vi "TimeLoop.vi"(4 "N":i32=100, 7 "Loop durations in":dbl[][](array[numeric])) -> (0 "Average fps":dbl, 3 "Loop durations out":dbl[][](array[numeric]))   [LabVIEW 2013]
doc: "Calculate average loop frequency over the last N (default: 100) iterations.\n\nMostly used for debugging"
uses:
  <vilib>/Analysis/baseanly.llb/Mean (DBL).vi
  <vilib>/Analysis/NI_AALBase.lvlib
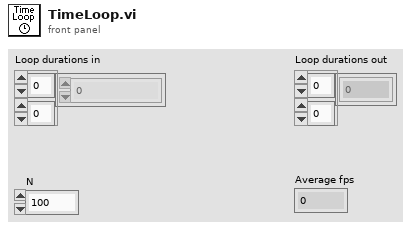
[diagram p1: front panel]
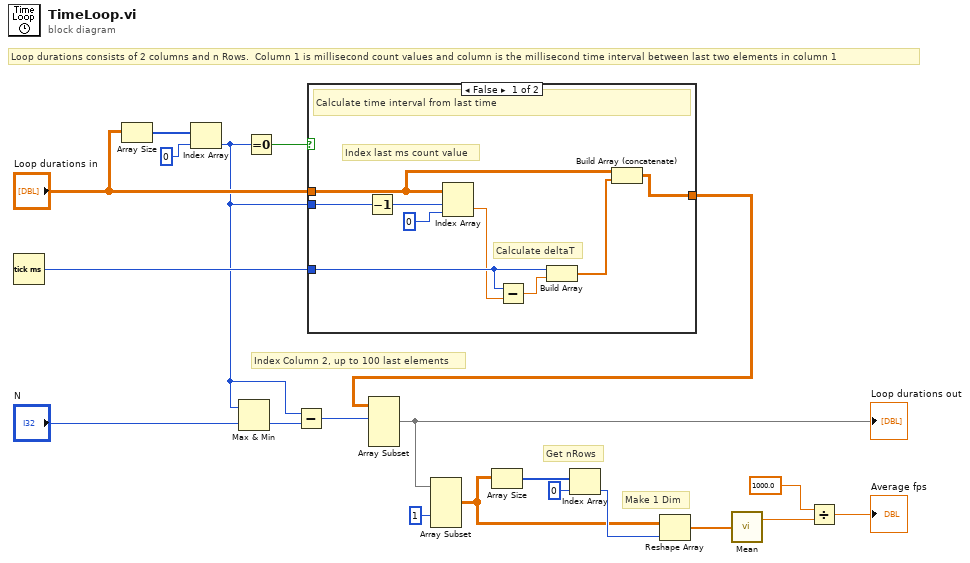
[diagram p0: block diagram]
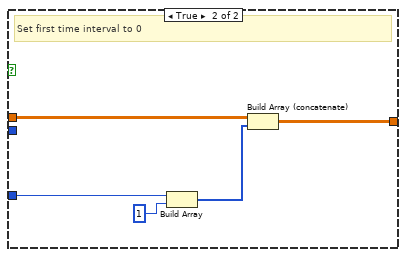
[diagram p2: hidden frame]
diagram:
  # "Get nRows"
  # "Loop durations consists of 2 columns and n Rows.  Column 1 is millisecond count values and column is the millisecond time interval between last two elements in column 1"
  # "Make 1 Dim"
  # "Index Column 2, up to 100 last elements"
  n1 = Tick Count (ms)() -> (millisecond timer value=w19:u32)
  n2 = Array Size(array="Loop durations in") -> (size(s)=w11:i32[])
  n3 = Index Array(array=w11, index=0) -> (element=w5:i32)
  n4 = Max & Min(x=w5, y="N") -> (min(x,y)=w6:i32)  [unwired: 1 out]
  n5 = Equal To 0?(x=w5) -> (x = 0?=w20:bool)
  n6 = Subtract(x=w5, y=w6) -> (x-y=w4:i32)
  n7 = case shown="False" w20 {
    tunnel: w19 -> [w26 w34]
    tunnel: "Loop durations in" -> [w28 w31]
    tunnel: [w27 w30] -> w17
    tunnel: w5 -> [w22 _]
    frame False {
      # "Calculate deltaT"
      # "Index last ms count value"
      # "Calculate time interval from last time"
      n8 = Decrement(x=w22) -> (x-1=w21:i32)
      n9 = Index Array(array=w28, index (row)=w21, index (col)=0 ("disabled index (col)")) -> (element=w25:dbl)
      n10 = Subtract(x=w26, y=w25) -> (x-y=w23:dbl)
      n11 = Build Array(w26, w23) -> (w29:dbl[])
      n12 = Build Array (concatenate)(w28, w29) -> (w27:dbl[][])
    }
    frame True {
      # "Set first time interval to 0"
      n13 = Build Array(w34, u32 1 ("element")) -> (w32:u32[])
      n14 = Build Array (concatenate)(w31, w32) -> (w30:dbl[][])
    }
  }
  n15 = Array Subset(array=w17, index (row)=w4) -> (w3:dbl[][])  [unwired: 3 in]
  "Loop durations out" <- w3
  n16 = Array Subset(array=w3, index (col)=1 ("index")) -> (w1:dbl[][])  [unwired: 3 in]
  n17 = Array Size(array=w1) -> (size(s)=w16:i32[])
  n18 = Index Array(array=w16, index=0) -> (element=w14:i32)
  n19 = Reshape Array(w1, w14) -> (w13:dbl[])
  n20 = call-poly <vilib>:"Mean.vi"("X"=w13) -> ("mean"=w10:dbl)  [unwired: 1 out]
  n21 = Divide(x=1000.0, y=w10) -> (x/y=→"Average fps":dbl)
